vi "mobility_subvi_07_13a_JW.vi"(8 "NumPts":dbl=5.0, 11 "Path":path) -> (0 "XY Graph-Sat":cluster{dbl[], dbl[]}[](graph), 1 "XY Graph-Lin":cluster{dbl[], dbl[]}[](graph), 3 "Output":T1, 4 "Index-Sat":dbl, 5 "Index-Lin":dbl)   [LabVIEW 2011]
uses:
  <vilib>/Utility/file.llb/Read From Spreadsheet File (string).vi
panel:
  out "Mobility-Lin":dbl
  out "Vt-Lin":dbl
  out "Lin Vd":dbl
  out "Vt-Sat":dbl
  out "Mobility-Sat":dbl
  out "Data Length":dbl
  out "Vg Column":dbl[](array[numeric])
  out "Saturation Id":dbl[](array[numeric])
  out "Linear Id":dbl[](array[numeric])
  out "File Array Length":dbl
  out "Data Array":string[][](array[string])
  out "Dielectric (d)":dbl
  out "Width":dbl
  out "Length":dbl
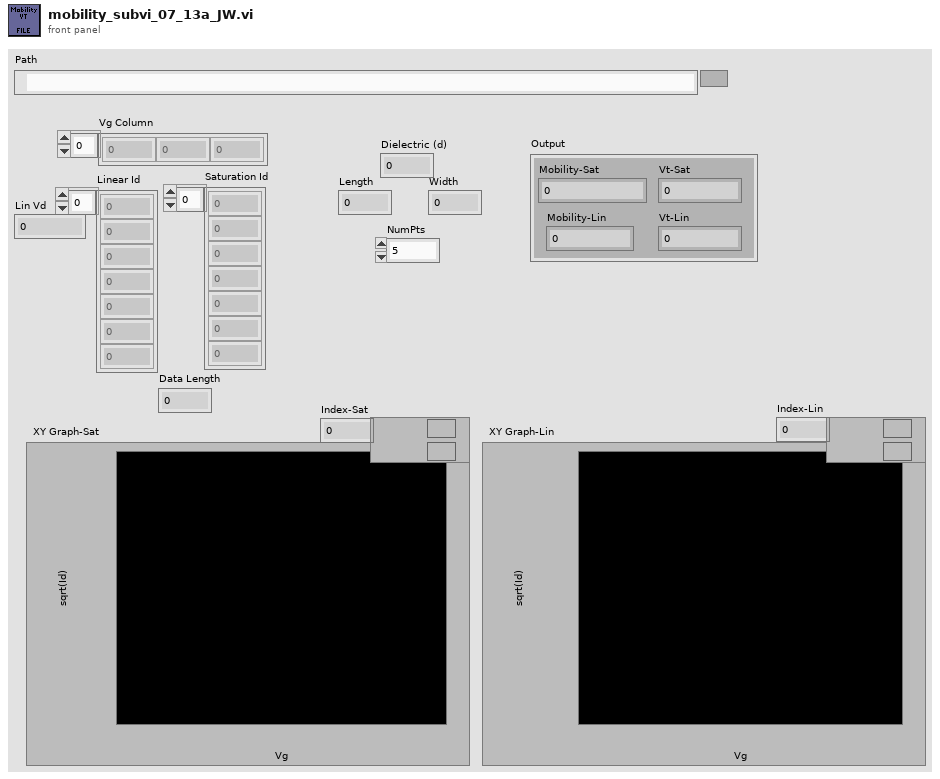
[diagram p1: front panel]
types:
  T1 = cluster{"Mobility-Sat":dbl, "Vt-Sat":dbl, "Mobility-Lin":dbl, "Vt-Lin":dbl}
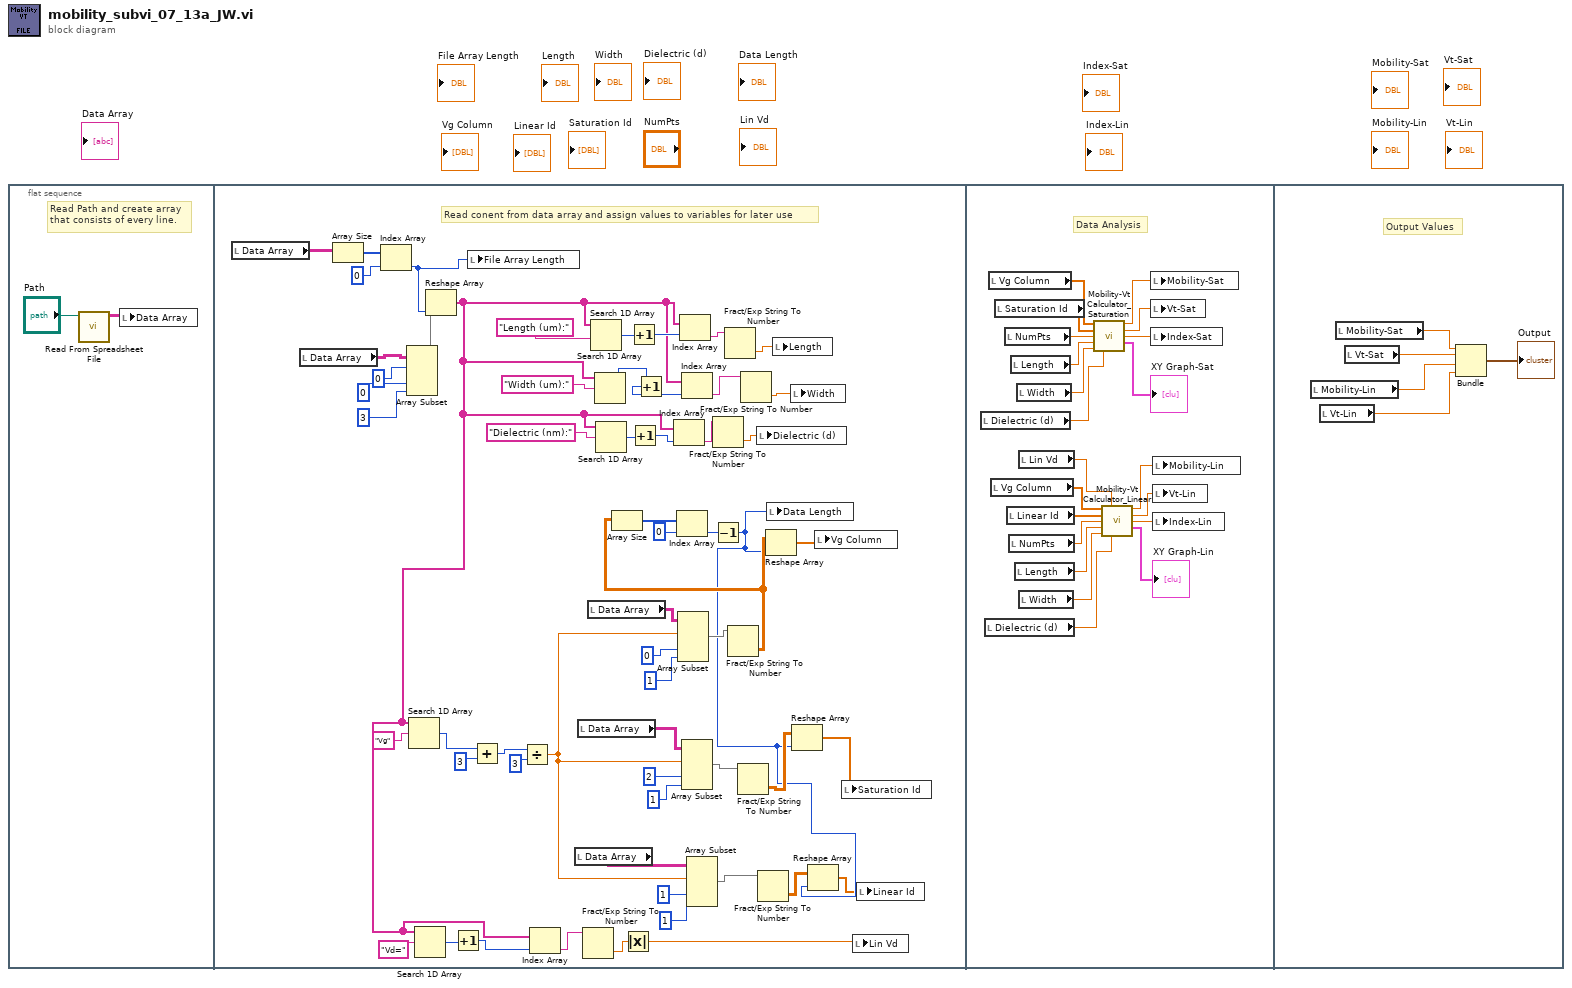
[diagram p0: block diagram]
diagram:
  n1 = flat-sequence {
    frame #0 {
      # "Read Path and create array\nthat consists of every line."
      n2 = call-poly <vilib>:"Read From Spreadsheet File.vi"("file path (dialog if empty)"="Path") -> ("all rows"=w2:string[][])  [unwired: 6 in, 4 out]
      n3 = local write "Data Array"(w2) -> ()
    }
    frame #1 {
      # "Read conent from data array and assign values to variables for later use"
      n4 = local read "Data Array"() -> (w41:string[][])
      n5 = local read "Data Array"() -> (w40:string[][])
      n6 = Array Size(array=w41) -> (size(s)=w61:i32[])
      n7 = Index Array(array=w61, index=0) -> (element=w34:i32)
      n8 = Array Subset(array=w40, index (row)=0, index (col)=0, length (col)=3) -> (w56:string[][])  [unwired: 1 in]
      n9 = Reshape Array(w56, w34) -> (w7:string[])
      n10 = Search 1D Array(1D array=w7, element="Vg") -> (index of element=w43:i32)  [unwired: 1 in]
      n11 = Search 1D Array(1D array=w7, element="Vd=") -> (index of element=w8:i32)  [unwired: 1 in]
      n12 = Increment(x=w8) -> (x+1=w6:i32)
      n13 = local write "File Array Length"(w34) -> ()
      n14 = Add(x=w43, y=3) -> (x+y=w45:i32)
      n15 = Divide(x=w45, y=3) -> (x/y=w21:dbl)
      n16 = Index Array(array=w7, index=w6) -> (element=w5:string)
      n17 = local read "Data Array"() -> (w23:string[][])
      n18 = local read "Data Array"() -> (w22:string[][])
      n19 = Fract/Exp String To Number(string=w5) -> (number=w3:dbl)  [unwired: 3 in, 1 out]
      n20 = local read "Data Array"() -> (w24:string[][])
      n21 = Search 1D Array(1D array=w7, element="Length (um):") -> (index of element=w52:i32)  [unwired: 1 in]
      n22 = Search 1D Array(1D array=w7, element="Width (um):") -> (index of element=w53:i32)  [unwired: 1 in]
      n23 = Search 1D Array(1D array=w7, element="Dielectric (nm):") -> (index of element=w48:i32)  [unwired: 1 in]
      n24 = Absolute Value(x=w3) -> (abs(x)=w4:dbl)
      n25 = Increment(x=w52) -> (x+1=w54:i32)
      n26 = Increment(x=w48) -> (x+1=w47:i32)
      n27 = Increment(x=w53) -> (x+1=w55:i32)
      n28 = Index Array(array=w7, index=w47) -> (element=w39:string)
      n29 = Array Subset(array=w24, index (row)=w21, index (col)=0, length (col)=1) -> (w26:string[][])  [unwired: 1 in]
      n30 = Index Array(array=w7, index=w54) -> (element=w35:string)
      n31 = Index Array(array=w7, index=w55) -> (element=w38:string)
      n32 = Array Subset(array=w22, index (row)=w21, index (col)=2, length (col)=1) -> (w25:string[][])  [unwired: 1 in]
      n33 = Array Subset(array=w23, index (row)=w21, index (col)=1, length (col)=1) -> (w11:string[][])  [unwired: 1 in]
      n34 = Fract/Exp String To Number(string=w39) -> (number=w33:dbl)  [unwired: 3 in, 1 out]
      n35 = Fract/Exp String To Number(string=w35) -> (number=w36:dbl)  [unwired: 3 in, 1 out]
      n36 = Fract/Exp String To Number(string=w26) -> (number=w16:dbl[][])  [unwired: 3 in, 1 out]
      n37 = Array Size(array=w16) -> (size(s)=w17:i32[])
      n38 = Index Array(array=w17, index=0) -> (element=w19:i32)
      n39 = Decrement(x=w19) -> (x-1=w12:i32)
      n40 = Fract/Exp String To Number(string=w25) -> (number=w15:dbl[][])  [unwired: 3 in, 1 out]
      n41 = Fract/Exp String To Number(string=w38) -> (number=w37:dbl)  [unwired: 3 in, 1 out]
      n42 = local write "Dielectric (d)"(w33) -> ()
      n43 = Fract/Exp String To Number(string=w11) -> (number=w13:dbl[][])  [unwired: 3 in, 1 out]
      n44 = Reshape Array(w16, w12) -> (w20:dbl[])
      n45 = local write "Data Length"(w12) -> ()
      n46 = local write "Length"(w36) -> ()
      n47 = local write "Width"(w37) -> ()
      n48 = Reshape Array(w15, w12) -> (w14:dbl[])
      n49 = Reshape Array(w13, w12) -> (w10:dbl[])
      n50 = local write "Vg Column"(w20) -> ()
      n51 = local write "Saturation Id"(w14) -> ()
      n52 = local write "Lin Vd"(w4) -> ()
      n53 = local write "Linear Id"(w10) -> ()
    }
    frame #2 {
      # "Data Analysis"
      n54 = local read "Dielectric (d)"() -> (w77:dbl)
      n55 = local read "Dielectric (d)"() -> (w67:dbl)
      n56 = local read "Vg Column"() -> (w82:dbl[])
      n57 = local read "Vg Column"() -> (w72:dbl[])
      n58 = local read "Saturation Id"() -> (w81:dbl[])
      n59 = local read "NumPts"() -> (w80:dbl)
      n60 = local read "Linear Id"() -> (w71:dbl[])
      n61 = local read "NumPts"() -> (w70:dbl)
      n62 = local read "Length"() -> (w79:dbl)
      n63 = local read "Length"() -> (w69:dbl)
      n64 = local read "Width"() -> (w78:dbl)
      n65 = local read "Lin Vd"() -> (w66:dbl)
      n66 = local read "Width"() -> (w68:dbl)
      n67 = call "Mobility-Vt Calculator_Saturation.vi"("Vg Column"=w82, "Sat Id Column"=w81, "NumPts"=w80, "Length"=w79, "Width"=w78, "Dielectric Thickness"=w77) -> ("Mobility-Sat"=w76:dbl, "VT-Sat"=w75:dbl, "Index-Sat"=w73:dbl, "XY Graph-Sat"=→"XY Graph-Sat":cluster{dbl[], dbl[]}[])  [unwired: 4 in, 2 out]
      n68 = call "Mobility-Vt Calculator_Linear.vi"("Vg Column"=w72, "Vd"=w66, "Lin Id Column"=w71, "NumPts"=w70, "Length"=w69, "Width"=w68, "Dielectric Thickness"=w67) -> ("Mobility-Lin"=w65:dbl, "VT-Lin"=w64:dbl, "Index-Lin"=w63:dbl, "LinSat"=→"XY Graph-Lin":cluster{dbl[], dbl[]}[])  [unwired: 5 in]
      n69 = local write "Mobility-Sat"(w76) -> ()
      n70 = local write "Vt-Sat"(w75) -> ()
      n71 = local write "Index-Sat"(w73) -> ()
      n72 = local write "Mobility-Lin"(w65) -> ()
      n73 = local write "Vt-Lin"(w64) -> ()
      n74 = local write "Index-Lin"(w63) -> ()
    }
    frame #3 {
      # "Output Values"
      n75 = local read "Mobility-Lin"() -> (w85:dbl)
      n76 = local read "Vt-Lin"() -> (w84:dbl)
      n77 = local read "Mobility-Sat"() -> (w87:dbl)
      n78 = local read "Vt-Sat"() -> (w86:dbl)
      n79 = Bundle("Mobility-Sat"=w87, "Vt-Sat"=w86, "Mobility-Lin"=w85, "Vt-Lin"=w84) -> (→"Output":T1)  [unwired: 1 in]
    }
  }
